vi "SetTriggerDelay.vi"(8 "Error In":errorcluster, 10 "Delay (sec)":dbl min=0.0 max=999.9999, 11 "Keithley 6482 In":refnum<visa-resource-name>) -> (0 "Error Out":errorcluster, 3 "Keithley 6482 Out":refnum<visa-resource-name>)   [LabVIEW 2014, in "Keithley-6482-Visa.lvlib"]
uses:
  Keithley-6482-Visa.lvlib
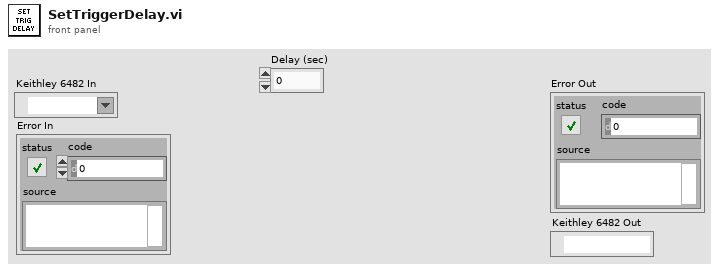
[diagram p1: front panel]
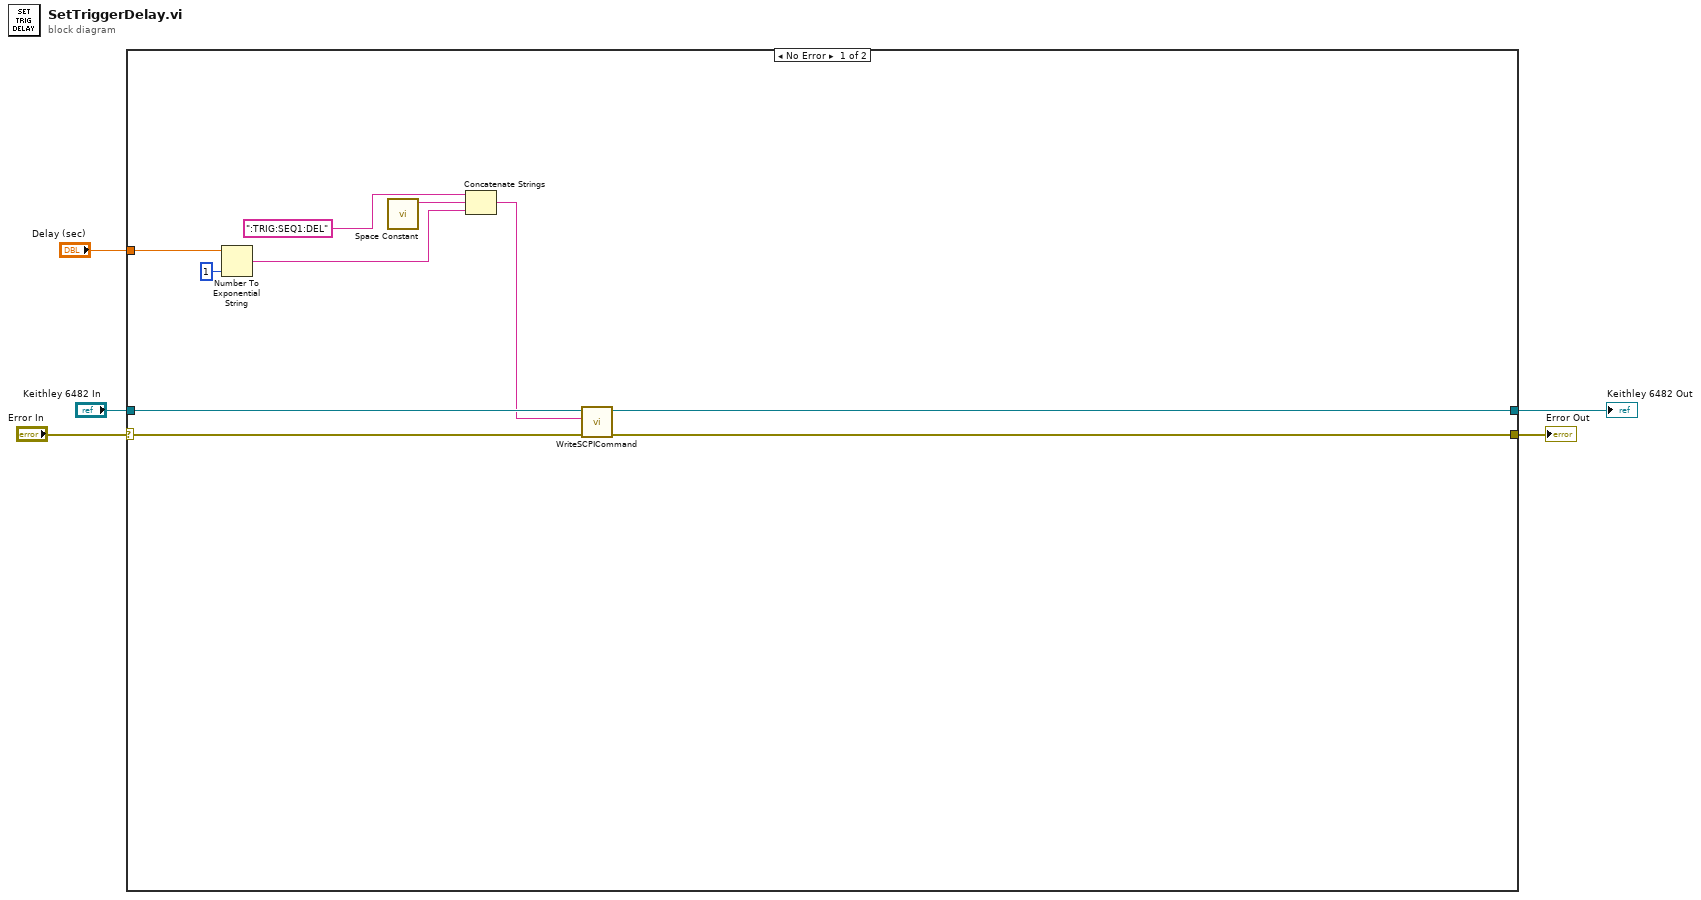
[diagram p0: block diagram]
diagram:
  n1 = case shown="No Error" "Error In" {
    selector: "Error In" -> [w15 w16]
    tunnel: "Keithley 6482 In" -> [w14 w17]
    tunnel: [w6 w16] -> w3
    tunnel: [w7 w17] -> w2
    tunnel: "Delay (sec)" -> [w11 _]
    frame No Error {
      n2 = Number To Exponential String(number=w11, precision (6)=i16 1) -> (E-format string=w9:string)  [unwired: 2 in]
      n3 = call <vilib>:"Space Constant.vi"() -> ("String"=w12:string)
      n4 = Concatenate Strings(":TRIG:SEQ1:DEL" ("string"), w12, w9) -> (w8:string)
      n5 = call "WriteSCPICommand.vi"("Error In"=w15, "SCPI Command"=w8, "Keithley 6482 In"=w14) -> ("Error Out"=w6:errorcluster, "Keithley 6482 Out"=w7:refnum<visa-resource-name>)  [unwired: 7 in]
    }
    frame Error {
    }
  }
  "Error Out" <- w3
  "Keithley 6482 Out" <- w2
